vi "assemble.vi"(8 "error in (no error)":errorcluster, 11 "IFurniture in":refnum<class "IFurniture.lvclass">) -> (0 "error out":errorcluster, 2 "String":string, 3 "IFurniture out":refnum<class "IFurniture.lvclass">)   [LabVIEW 2021, in "IFurniture.lvclass"]
uses:
  IFurniture.lvclass
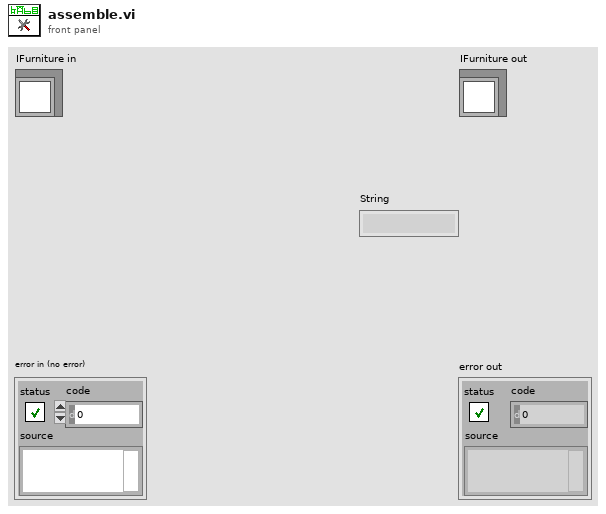
[diagram p1: front panel]
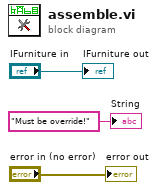
[diagram p0: block diagram]
diagram:
  "error out" <- "error in (no error)"
  "IFurniture out" <- "IFurniture in"
  "String" <- "Must be override!" ("String")
